vi "Synchronize.vi"(8 "error in (no error)":errorcluster, 11 "SCADA in":refnum<class "SCADA.lvclass">) -> (0 "error out":errorcluster, 3 "SCADA out":refnum<class "SCADA.lvclass">)   [LabVIEW 2015, in "SCADA Core.lvlib" / "SCADA.lvclass"]
uses:
  SCADA.lvclass
  SCADA.lvclass/SCADA.ctl
  <vilib>/ActorFramework/Message Enqueuer/Message Enqueuer.lvclass/Message Enqueuer.ctl
  IED Actor/IED Messages/Synchronize Msg/Synchronize Msg.lvclass/Synchronize Msg.ctl
  SCADA Abstract Messages/Simple Command Status Msg/Simple Command Status.ctl
  <vilib>/ActorFramework/Actor/Actor.lvclass/Actor.ctl
  <vilib>/Utility/error.llb/DialogType.ctl
  SCADA Response Messages/Return Synchronize Status Msg/Return Synchronize Status Msg.lvclass/Return Synchronize Status Msg.ctl
  <vilib>/ActorFramework/Message Enqueuer/Enqueue.vi
  <vilib>/ActorFramework/Message Enqueuer/Init from Existing Queue.vi
  <vilib>/ActorFramework/Message Priority Queue/Priority Enqueue.vi
  IED Actor/IED Messages/Ready Frequency Control for Sync Msg/Ready Frequency Control for Sync Msg.lvclass
  IED Actor/IED Messages/Synchronize Msg/Synchronize Msg.lvclass
  <vilib>/ActorFramework/Message Enqueuer/Message Enqueuer.lvclass
  SCADA Response Messages/Return Synchronize Status Msg/Return Synchronize Status Msg.lvclass
  SCADA Abstract Messages/Simple Command Status Msg/Simple Command Status Msg.lvclass
  <vilib>/ActorFramework/Actor/Actor.lvclass
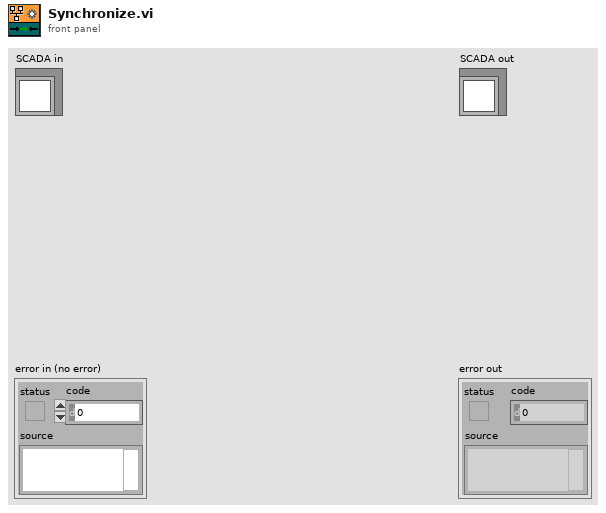
[diagram p1: front panel]
types:
  T1 = typedef "SCADA Core.lvlib/Simple Command Status Msg.lvclass/Simple Command Status.ctl" = enum16{"Success", "Failure"}
  T2 = typedef "SCADA Core.lvlib/SCADA.lvclass/Grid Mode.ctl" = enum16{"Off", "Grid Connected", "Islanded", "Synchronizing"}
  T3 = typedef "DialogType.ctl" = u16
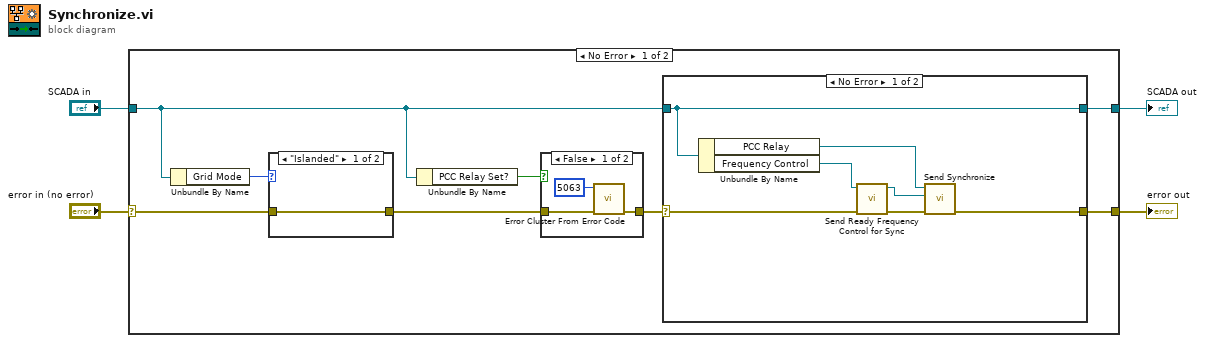
[diagram p0: block diagram]
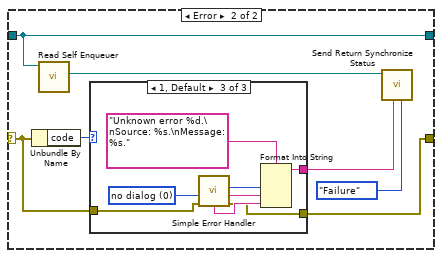
[diagram p2: hidden frame]
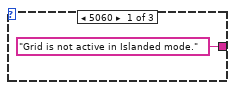
[diagram p3: hidden frame]
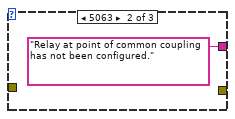
[diagram p4: hidden frame]
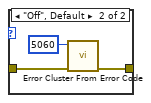
[diagram p6: hidden frame]
diagram:
  n1 = case shown="No Error" "error in (no error)" {
    selector: "error in (no error)" -> [w11 w46]
    tunnel: [w6 w46] -> w3
    tunnel: [w7 w45] -> w1
    tunnel: "SCADA in" -> [w8 w45]
    frame No Error {
      n2 = Unbundle By Name(w8) -> ("Grid Mode"=w12:T2)
      n3 = case shown="\"Islanded\"" w12 {
        tunnel: w11 -> [w41 w44]
        tunnel: [w41 w42] -> w5
        frame "Islanded" {
        }
        frame "Off", Default {
          n4 = call <vilib>:"Error Cluster From Error Code.vi"("error in (no error)"=w44, "error code (0)"=5060) -> ("error out"=w42:errorcluster)  [unwired: 7 in]
        }
      }
      n5 = Unbundle By Name(w8) -> ("PCC Relay Set?"=w10:bool)
      n6 = case shown="False" w10 {
        tunnel: w5 -> [w39 w40]
        tunnel: [w37 w40] -> w9
        frame False {
          n7 = call <vilib>:"Error Cluster From Error Code.vi"("error in (no error)"=w39, "error code (0)"=5063) -> ("error out"=w37:errorcluster)  [unwired: 7 in]
        }
        frame True {
        }
      }
      n8 = case shown="No Error" w9 {
        selector: w9 -> [w16 w25]
        tunnel: w8 -> [w19 w24]
        tunnel: [w19 w24] -> w7
        tunnel: [w17 w23] -> w6
        frame No Error {
          n9 = Unbundle By Name(w19) -> ("PCC Relay"=w18:refnum<class "Message Enqueuer.lvclass">, "Frequency Control"=w15:refnum<class "Message Enqueuer.lvclass">)
          n10 = call "Send Ready Frequency Control for Sync.vi"("error in (no error)"=w16, "Message Enqueuer"=w15) -> ("error out"=w13:errorcluster, "Message Enqueuer out"=w14:refnum<class "Message Enqueuer.lvclass">)  [unwired: 8 in]
          n11 = call "Send Synchronize.vi"("error in (no error)"=w13, "Frequency Control"=w14, "Message Enqueuer"=w18) -> ("error out"=w17:errorcluster)  [unwired: 7 in, 1 out]
        }
        frame Error {
          n12 = Unbundle By Name(w25) -> ("code"=w26:i32)
          n13 = call <vilib>:"Read Self Enqueuer.vi"("Actor"=w24) -> ("Self Enqueuer"=w22:refnum<class "Message Enqueuer.lvclass">)  [unwired: 10 in]
          n14 = case shown="1, Default" w26 {
            tunnel: w25 -> [_ _ w31]
            tunnel: ["Grid is not active in Islanded mode." "Relay at point of common coupling has not been configured." w30] -> w21
            tunnel: [_ _ w29] -> w23
            frame 5060 {
            }
            frame 5063 {
            }
            frame 1, Default {
              w32 = T3 0 items=["no dialog", "OK message", "continue or stop message", "OK message + warnings", "continue/stop + warnings"] ("type of dialog (OK msg:1)")
              n15 = call <vilib>:"Simple Error Handler.vi"("type of dialog (OK msg:1)"=w32, "error in (no error)"=w31) -> ("code out"=w34:i32, "source out"=w35:string, "error out"=w29:errorcluster, "message"=w36:string)  [unwired: 3 in, 1 out]
              n16 = Format Into String(format string="Unknown error %d.\nSource: %s.\nMessage: %s." ("Error String"), w34, w35, w36) -> (resulting string=w30:string)  [unwired: 2 in, 1 out]
            }
          }
          n17 = call "Send Return Synchronize Status.vi"("Status"=Simple_Command_Status."Failure", "error"=w21, "Message Enqueuer"=w22) -> ()  [unwired: 7 in, 2 out]
        }
      }
    }
    frame Error {
    }
  }
  "error out" <- w3
  "SCADA out" <- w1
